vi "FTW-Subscription-Construct.vi"(5 "Address":string, 11 "error in":errorcluster) -> (4 "FTW-Subscription Out":refnum<class "FTW-Subscription.lvclass">, 6 "Event Registration Refnum":refnum<event-registration>, 15 "error out":errorcluster)   [LabVIEW 2013, in "FTW-Subscription.lvclass"]
uses:
  FTW-Subscription.lvclass
  Message/Base/FTW-Message.lvclass
  Ether/FTW-Ether-EndpointType.ctl
  Endpoint/FTW-Endpoint.lvclass
  FTW-Subscription.lvclass/FTW-Subscription.ctl
  Ether/FTW-Ether.lvclass
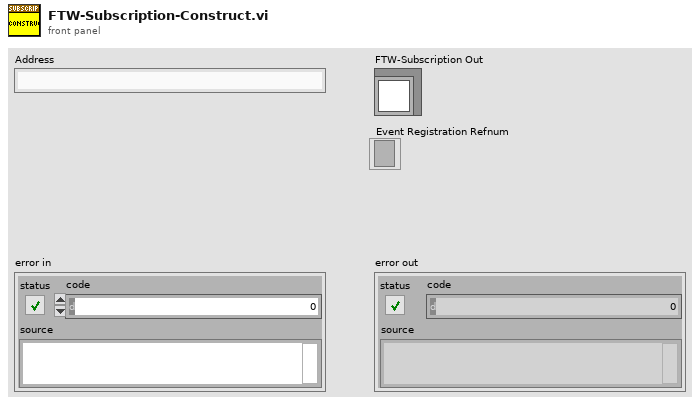
[diagram p1: front panel]
types:
  T1 = typedef "FTW-Ether.lvclass/FTW-Ether-EndpointType.ctl" = enum16{"Server", "Client", "Publisher", "Subscriber"}
  T2 = typedef "FTW-Ether.lvclass/FTW-Ether-MessageTransportScheme.ctl" = enum16{"LabVIEW Queues (lvq://)", "TCP (tcp://)", "LabVIEW Network Streams (lvns://)"}
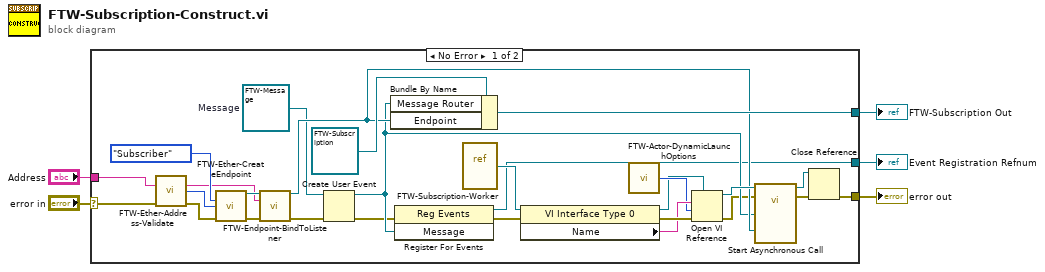
[diagram p0: block diagram]
diagram:
  n1 = case shown="No Error" "error in" {
    selector: "error in" -> [w6 w33]
    tunnel: [w10 w33] -> w4
    tunnel: [w24 _] -> w3
    tunnel: [w21 _] -> w1
    tunnel: "Address" -> [w16 _]
    frame No Error {
      w17 = refnum<class "FTW-Message.lvclass"> refnum  # Message
      n2 = call "FTW-Ether-Address-Validate.vi"("Address"=w16, "error in"=w6) -> ("Sanitized Address"=w12:string, "Message Transport Scheme"=w15:T2, "error out"=w13:errorcluster)  [unwired: 11 in]
      n3 = call "FTW-Ether-CreateEndpoint.vi"("Endpoint Type"=FTW-Ether-EndpointType."Subscriber", "Message Transport Scheme"=w15, "error in"=w13) -> ("FTW Endpoint"=w19:refnum<class "FTW-Endpoint.lvclass">, "error out"=w18:errorcluster)  [unwired: 11 in]
      n4 = call-dynamic "FTW-Endpoint-BindToListener.vi"("FTW-Endpoint In"=w19, "Address"=w12, "error in"=w18) -> ("FTW-Endpoint Out"=w23:refnum<class "FTW-Endpoint.lvclass">, "error out"=w7:errorcluster)  [unwired: 10 in, 1 out]
      n5 = Create User Event(user event datatype=w17, error in=w7) -> (user event=w22:refnum<user-event>, error out=w9:errorcluster)
      n6 = Bundle By Name(cluster=refnum<class "FTW-Subscription.lvclass"> refnum ("LVmsg_Router.lvclass"), "Message Router"=w22, "Endpoint"=w23) -> (w24:refnum<class "FTW-Subscription.lvclass">)
      n7 = register-events(error in=w9, w22) -> (reference out=w21:refnum<event-registration>, error out=w8:errorcluster)  [unwired: 1 in]
      n8 = vi-ref "FTW-Subscription-Worker.vi"() -> (w32:refnum<vi>)
      n9 = property class="VI Interface Type 0"(reference=w32, error in=w8) -> (reference out=w28:refnum<vi>, error out=w31:errorcluster, "Name"=w30:string)
      n10 = call "FTW-Actor-DynamicLaunchOptions.vi"() -> ("Open VI Ref Options"=w29:i32)
      n11 = Open VI Reference(type specifier VI Refnum (for type only)=w28, vi path=w30, options=w29, error in (no error)=w31) -> (vi reference=w26:refnum<vi>, error out=w11:errorcluster)  [unwired: 2 in]
      n12 = call-by-ref "Start Asynchronous Call"(reference=w26, error in=w11, "Socket"=w23, "Message Handler"=w22) -> (reference out=w20:refnum<vi>, error out=w27:errorcluster)  [unwired: 1 in]
      n13 = Close Reference(reference=w20, error in (no error)=w27) -> (error out=w10:errorcluster)
    }
    frame Error {
    }
  }
  "FTW-Subscription Out" <- w3
  "error out" <- w4
  "Event Registration Refnum" <- w1
